vi "Read and Update ERD Example.vi"(0 "GEA Inputs":T2 {"Destination" format="%.0x"; "Source" format="%.0x"}, 1 "Retry Count":i32=5, 2 "Read Timeout (ms)":u32=500, 5 "ERD Number":u16 format="%.0x", 7 "Update Information":string, 9 "Device Selected":i32, 11 "Error In":errorcluster, 13 "Verify ERD Response?":bool) -> (4 "Updated ERD Data Out":T1 {"ERD Number" format="%.0x"}, 6 "Updated Raw Data Out":string, 15 "Error Out":errorcluster)   [LabVIEW 2014]
doc: "This VI demonstrates the usage of the read and update ERD core functionality."
uses:
  type defs/Source_Destination.ctl
  type defs/ERD Read Data Out.ctl
  library/GEA2_Toolkit.lvlib
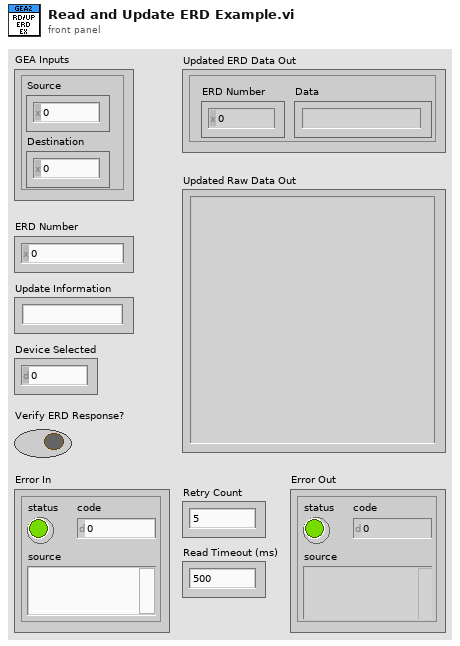
[diagram p1: front panel]
types:
  T1 = typedef "GEA2_Toolkit.lvlib/ERD Read Data Out.ctl" = cluster{"ERD Number":u16, "Data":string}
  T2 = typedef "GEA2_Toolkit.lvlib/Source_Destination.ctl" = cluster{"Source":u8, "Destination":u8}
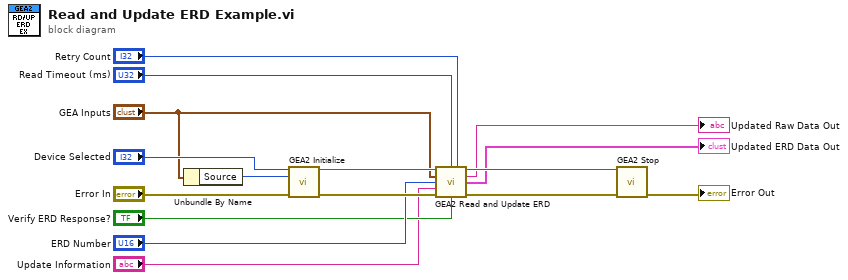
[diagram p0: block diagram]
diagram:
  n1 = Unbundle By Name("GEA Inputs") -> ("Source"=w13:u8)
  n2 = call "GEA2 Initialize.vi"("Board Index"="Device Selected", "Source Address"=w13, "error in"="Error In") -> ("GEA2 Reference Out"=w12:refnum<k24>, "error out"=w10:errorcluster)  [unwired: 10 in, 1 out]
  n3 = call "GEA2 Read and Update ERD.vi"("GEA2 Reference In"=w12, "Read Timeout (ms)"="Read Timeout (ms)", "Retry Count"="Retry Count", "GEA Inputs"="GEA Inputs", "ERD Number"="ERD Number", "Update Information"="Update Information", "Error In"=w10, "Verify ERD Response?"="Verify ERD Response?") -> ("GEA2 Reference Out"=w11:refnum<k24>, "Updated Raw Data Out"=→"Updated Raw Data Out":string, "Updated ERD Data Out"=→"Updated ERD Data Out":T1, "Error Out"=w9:errorcluster)  [unwired: 4 in]
  n4 = call "GEA2 Stop.vi"("GEA2 Reference In"=w11, "Error In"=w9) -> ("Error Out"=→"Error Out":errorcluster)  [unwired: 13 in]
